vi "Color_Result_Fixture.vi"(4 "Fixture_Data":u16[](array[numeric])) -> (1 "Array_Color_Result":u32[](array[numeric]))   [LabVIEW 2017]
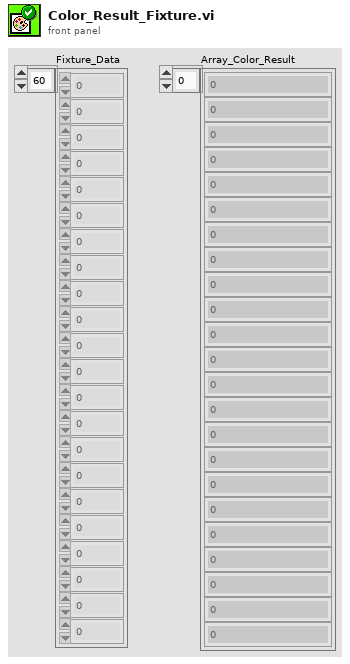
[diagram p1: front panel]
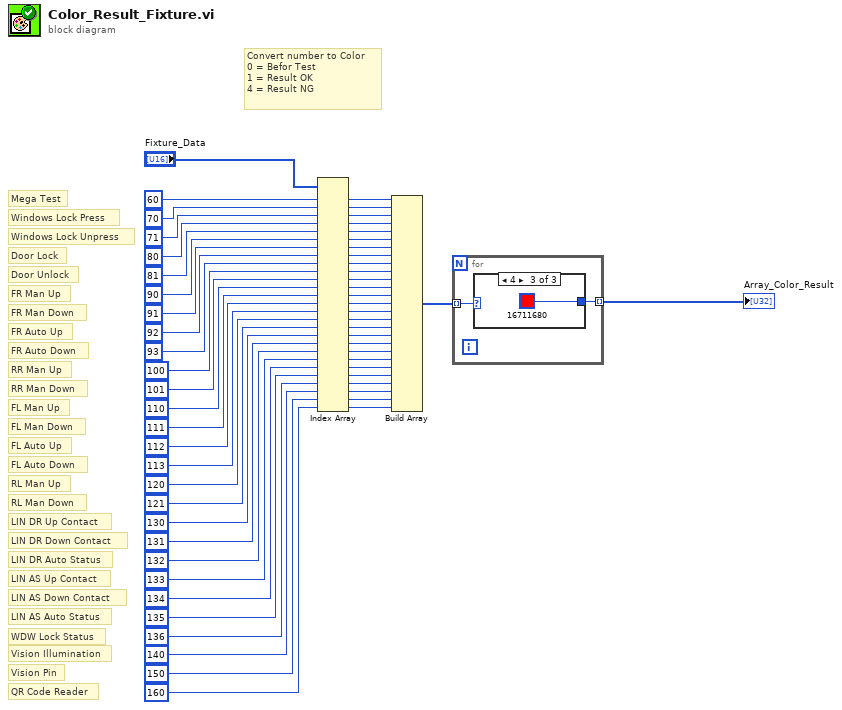
[diagram p0: block diagram]
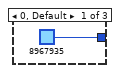
[diagram p2: hidden frame]
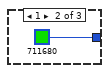
[diagram p3: hidden frame]
diagram:
  # "WDW Lock Status"
  # "QR Code Reader"
  # "Vision Pin"
  # "Vision Illumination"
  # "LIN AS Auto Status"
  # "LIN AS Down Contact"
  # "LIN AS Up Contact"
  # "LIN DR Auto Status"
  # "LIN DR Down Contact"
  # "LIN DR Up Contact"
  # "RL Man Down"
  # "RL Man Up"
  # "FL Auto Down"
  # "FL Auto Up"
  # "FL Man Down"
  # "FL Man Up"
  # "RR Man Down"
  # "RR Man Up"
  # "FR Auto Down"
  # "FR Auto Up"
  # "FR Man Down"
  # "FR Man Up"
  # "Door Unlock"
  # "Door Lock"
  # "Windows Lock Unpress"
  # "Windows Lock Press"
  # "Mega Test"
  # "Convert number to Color\n0 = Befor Test\n1 = Result OK\n4 = Result NG"
  n1 = Index Array(array="Fixture_Data", index #1=60 ("index"), index #2=70 ("index"), index #3=71 ("index"), index #4=80 ("index"), index #5=81 ("index"), index #6=90 ("index"), index #7=91 ("index"), index #8=92 ("index"), index #9=93 ("index"), index #10=100 ("index"), index #11=101 ("index"), index #12=110 ("index"), index #13=111 ("index"), index #14=112 ("index"), index #15=113 ("index"), index #16=120 ("index"), index #17=121 ("index"), index #18=130 ("index"), index #19=131 ("index"), index #20=132 ("index"), index #21=133 ("index"), index #22=134 ("index"), index #23=135 ("index"), index #24=136 ("index"), index #25=140 ("index"), index #26=150 ("index"), index #27=160 ("index")) -> (element #1=w56:u16, element #2=w54:u16, element #3=w50:u16, element #4=w49:u16, element #5=w48:u16, element #6=w29:u16, element #7=w28:u16, element #8=w27:u16, element #9=w26:u16, element #10=w25:u16, element #11=w24:u16, element #12=w23:u16, element #13=w22:u16, element #14=w21:u16, element #15=w20:u16, element #16=w19:u16, element #17=w18:u16, element #18=w17:u16, element #19=w16:u16, element #20=w15:u16, element #21=w14:u16, element #22=w13:u16, element #23=w12:u16, element #24=w11:u16, element #25=w10:u16, element #26=w9:u16, element #27=w1:u16)
  n2 = Build Array(w56, w54, w50, w49, w48, w29, w28, w27, w26, w25, w24, w23, w22, w21, w20, w19, w18, w17, w16, w15, w14, w13, w12, w11, w10, w9, w1) -> (w7:u16[])
  n3 = for {
    tunnel: w7 -> [w59] mode=indexing
    tunnel: [w58] -> w8 mode=indexing
    n4 = case shown="4" w59 {
      tunnel: [u32 8967935 u32 711680 u32 16711680] -> w58
      frame 0, Default {
      }
      frame 1 {
      }
      frame 4 {
      }
    }
  }
  "Array_Color_Result" <- w8
